vi "8.steper-motor.vi"() -> ()   [LabVIEW 2011]
panel:
  out "Waveform Graph 3":dynamicdata(graph)
  out "Waveform Graph 2":dynamicdata(graph)
  out "Waveform Graph":dynamicdata(graph)
  in  "frequency":dbl
  out "Waveform Graph":dynamicdata(graph)
  in  "stop":bool
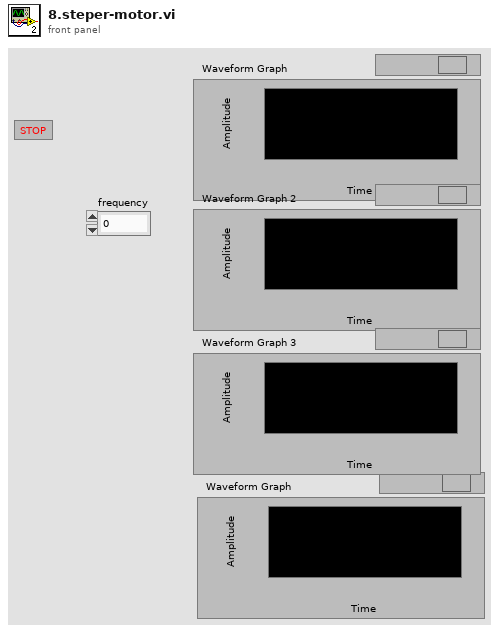
[diagram p1: front panel]
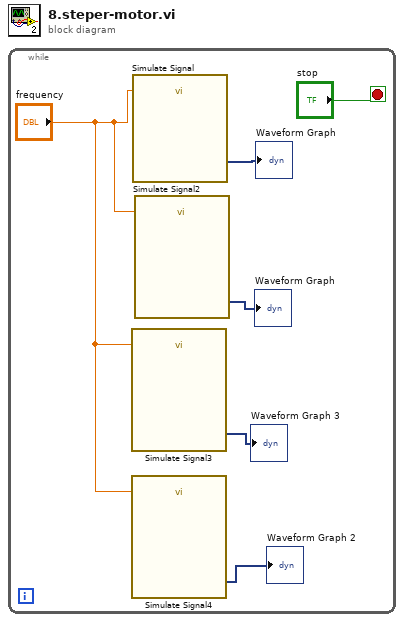
[diagram p0: block diagram]
diagram:
  n1 = while {
    stop <- "stop" stop-if-true
    n2 = call "Simulate Signal3"("Frequency"="frequency") -> ("Square"=→"Waveform Graph 3":dynamicdata)  [unwired: 13 in, 1 out]
    n3 = call "Simulate Signal4"("Frequency"="frequency") -> ("Square"=→"Waveform Graph 2":dynamicdata)  [unwired: 13 in, 1 out]
    n4 = call "Simulate Signal"("Frequency"="frequency") -> ("Square"=→"Waveform Graph":dynamicdata)  [unwired: 13 in, 1 out]
    n5 = call "Simulate Signal2"("Frequency"="frequency") -> ("Square"=→"Waveform Graph":dynamicdata)  [unwired: 13 in, 1 out]
  }
